vi "Create Event References.vi"(8 "error in (no error)":errorcluster, 11 "Engine in":refnum<class "Engine.lvclass">) -> (0 "error out":errorcluster, 3 "Engine out":refnum<class "Engine.lvclass">)   [LabVIEW 2023, in "Engine.lvlib" / "Engine.lvclass"]
doc: "This routine creates events references. It should only be called when the initialization being performed is the root actor. (<b>IsRoot == TRUE</b>)"
uses:
  Project/Engine.lvclass
  Custom Controls/System Status.ctl
  Project/Engine.lvclass/Engine.ctl
  builds/Tools/QDMH.lvlibp/QDMH.lvclass
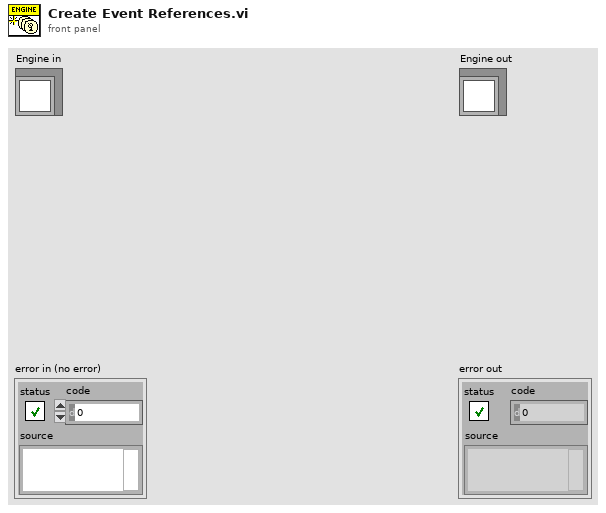
[diagram p1: front panel]
types:
  T1 = typedef "Engine.lvlib/Engine.lvclass/System Status.ctl" = enum16{"Logged Off", "UUT_Info_Missing", "Idle", "Error", "Warning", "Loading", "Config", "Manual", "Automation", "Report_View", "Previous"}
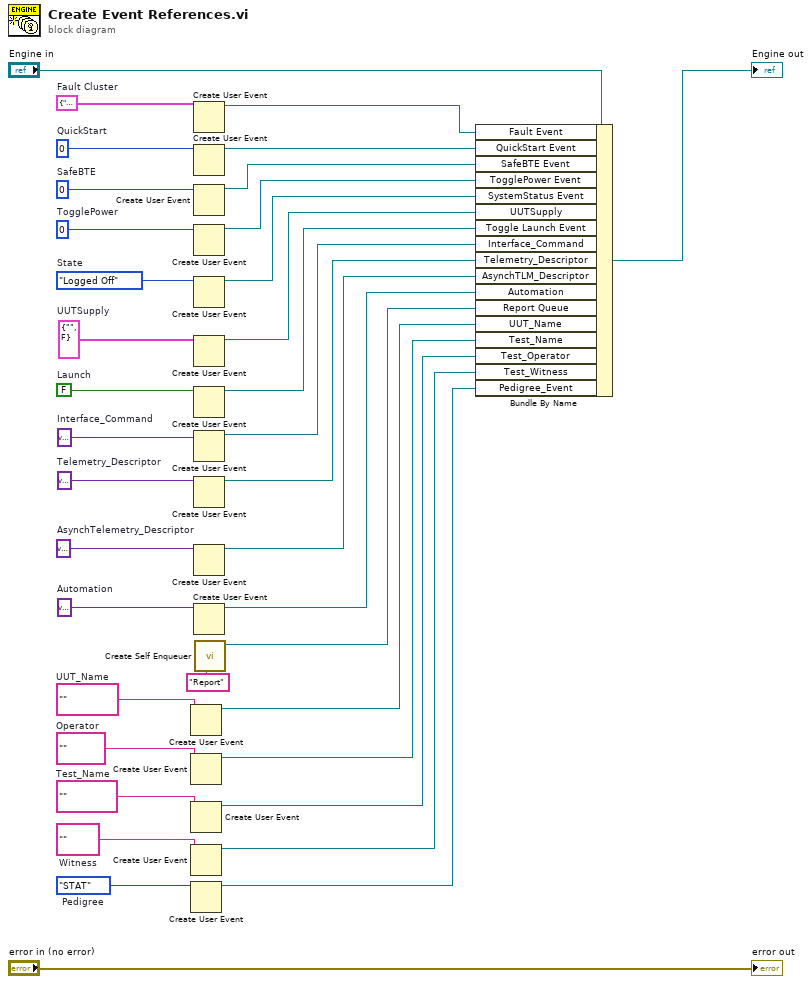
[diagram p0: block diagram]
diagram:
  w1 = cluster{"Source":string, "Fault":errorcluster} {"Source"="", "Fault"={"status"=FALSE, "code"=0, "source"=""}}  # Fault Cluster
  w11 = enum16{"STAT", "BB", "PT", "EM", "FT"}."STAT"  # Pedigree
  w10 = ""  # Witness
  w9 = ""  # Test_Name
  w8 = ""  # Operator
  w7 = ""  # UUT_Name
  w14 = System_Status."Logged Off"  # State
  w30 = variant  # Automation
  w29 = variant  # AsynchTelemetry_Descriptor
  w28 = variant  # Telemetry_Descriptor
  w27 = variant  # Interface_Command
  w26 = FALSE  # Launch
  w31 = cluster{"Supply":string, "Output":bool} {"Supply"="", "Output"=FALSE}  # UUTSupply
  w34 = 0  # TogglePower
  w33 = 0  # SafeBTE
  w32 = 0  # QuickStart
  n1 = Create User Event(user event datatype=w7) -> (user event=w6:refnum<user-event>)  [unwired: 1 in, 1 out]
  n2 = Create User Event(user event datatype=w8) -> (user event=w5:refnum<user-event>)  [unwired: 1 in, 1 out]
  n3 = Create User Event(user event datatype=w9) -> (user event=w4:refnum<user-event>)  [unwired: 1 in, 1 out]
  n4 = Create User Event(user event datatype=w10) -> (user event=w3:refnum<user-event>)  [unwired: 1 in, 1 out]
  n5 = Create User Event(user event datatype=w11) -> (user event=w2:refnum<user-event>)  [unwired: 1 in, 1 out]
  n6 = Create User Event(user event datatype=w1) -> (user event=w25:refnum<user-event>)  [unwired: 1 in, 1 out]
  n7 = Create User Event(user event datatype=w32) -> (user event=w24:refnum<user-event>)  [unwired: 1 in, 1 out]
  n8 = Create User Event(user event datatype=w33) -> (user event=w23:refnum<user-event>)  [unwired: 1 in, 1 out]
  n9 = Create User Event(user event datatype=w34) -> (user event=w22:refnum<user-event>)  [unwired: 1 in, 1 out]
  n10 = Create User Event(user event datatype=w14) -> (user event=w21:refnum<user-event>)  [unwired: 1 in, 1 out]
  n11 = Create User Event(user event datatype=w31) -> (user event=w20:refnum<user-event>)  [unwired: 1 in, 1 out]
  n12 = Create User Event(user event datatype=w26) -> (user event=w19:refnum<user-event>)  [unwired: 1 in, 1 out]
  n13 = Create User Event(user event datatype=w27) -> (user event=w18:refnum<user-event>)  [unwired: 1 in, 1 out]
  n14 = Create User Event(user event datatype=w28) -> (user event=w17:refnum<user-event>)  [unwired: 1 in, 1 out]
  n15 = Create User Event(user event datatype=w29) -> (user event=w16:refnum<user-event>)  [unwired: 1 in, 1 out]
  n16 = Create User Event(user event datatype=w30) -> (user event=w15:refnum<user-event>)  [unwired: 1 in, 1 out]
  n17 = call "Create Self Enqueuer.vi"("Name"="Report") -> ("QDMH out"=w12:refnum<class "QDMH.lvclass">)  [unwired: 9 in, 1 out]
  n18 = Bundle By Name(cluster="Engine in", "Fault Event"=w25, "QuickStart Event"=w24, "SafeBTE Event"=w23, "TogglePower Event"=w22, "SystemStatus Event"=w21, "UUTSupply"=w20, "Toggle Launch Event"=w19, "Interface_Command"=w18, "Telemetry_Descriptor"=w17, "AsynchTLM_Descriptor"=w16, "Automation"=w15, "Report Queue"=w12, "UUT_Name"=w6, "Test_Name"=w5, "Test_Operator"=w4, "Test_Witness"=w3, "Pedigree_Event"=w2) -> (→"Engine out":refnum<class "Engine.lvclass">)
  "error out" <- "error in (no error)"
